vi "3darray to cluster of 2d.vi"(11 "Array":dbl[][][](array[numeric])) -> (3 "Cluster":T1)   [LabVIEW 2017]
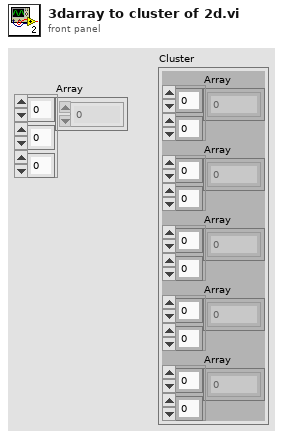
[diagram p1: front panel]
types:
  T1 = cluster{"Array":dbl[][], "Array":dbl[][], "Array":dbl[][], "Array":dbl[][], "Array":dbl[][]}
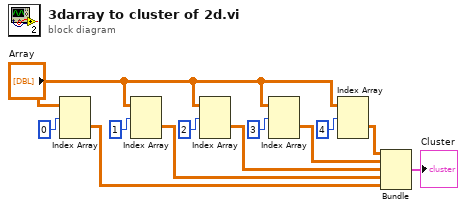
[diagram p0: block diagram]
diagram:
  n1 = Index Array(array="Array", index (dim 0)=0 ("index (page)")) -> (element=w12:dbl[][])  [unwired: 2 in]
  n2 = Index Array(array="Array", index (dim 0)=1 ("index (page)")) -> (element=w11:dbl[][])  [unwired: 2 in]
  n3 = Index Array(array="Array", index (dim 0)=2 ("index (page)")) -> (element=w10:dbl[][])  [unwired: 2 in]
  n4 = Index Array(array="Array", index (dim 0)=3 ("index (page)")) -> (element=w9:dbl[][])  [unwired: 2 in]
  n5 = Index Array(array="Array", index (dim 0)=4 ("index (page)")) -> (element=w8:dbl[][])  [unwired: 2 in]
  n6 = Bundle("Array"=w8, "Array"=w9, "Array"=w10, "Array"=w11, "Array"=w12) -> (→"Cluster":T1)  [unwired: 1 in]
